vi "SaveTrendData.vi"(6 "registry":T9, 8 "error in (no error)":errorcluster, 9 "data":T13, 10 "data event config":T17, 11 "data event":T1) -> (0 "error out":errorcluster, 3 "data event out":T1)   [LabVIEW 2017, in "EmsaDataEventCreator.lvlib"]
uses:
  <vilib>/addons/InsightCM/Devices/Shared/Emsa/EmsaDataEventCreator/EmsaDataEventCreator.lvlib
  <vilib>/addons/InsightCM/Devices/Shared/Emsa/EmsaDataEventCreator/controls/DataEventConfig.ctl
  <vilib>/addons/PointValueMap/controls/PointMap.ctl
  <vilib>/addons/InsightCM/Devices/Shared/Emsa/EmsaDataEventCreator/controls/SweepParams.ctl
  <vilib>/addons/InsightCM/Devices/Shared/Common/DataFlow/controls/Data.ctl
  <vilib>/addons/InsightCM/Utilities/DataAccessors/controls/wfmSGL_DVR.ctl
  <vilib>/addons/InsightCM/Devices/Shared/Common/DataFlow/controls/Type.ctl
  <vilib>/addons/InsightCM/Devices/Shared/Emsa/EmsaDataEventCreator/controls/Registry.ctl
  <vilib>/addons/InsightCM/Devices/Shared/Emsa/EmsaDataEventCreator/controls/Registry_Sweep.ctl
  <vilib>/addons/InsightCM/Devices/Shared/Common/DataEvent/controls/DataSetType.ctl
  <vilib>/addons/InsightCM/MessageBus/Base/controls/KeyValuePair.ctl
  <vilib>/addons/InsightCM/Devices/Shared/Common/DataEventCreator/controls/Registry_Trend.ctl
  <vilib>/addons/InsightCM/Devices/Shared/Common/DataEvent/controls/Event.ctl
  <vilib>/addons/InsightCM/MessageBus/Base/controls/DataEvent.ctl
  <vilib>/addons/InsightCM/Devices/Shared/Common/DataEvent/controls/DataSet.ctl
  <vilib>/addons/InsightCM/MessageBus/Base/controls/DataSetMetadata.ctl
  <vilib>/addons/InsightCM/MessageBus/Base/controls/TrendPoint.ctl
  <vilib>/addons/InsightCM/MessageBus/Base/controls/TrendAlarmUpdate.ctl
  <vilib>/addons/InsightCM/MessageBus/Base/controls/TrendAlarmTransition.ctl
  <vilib>/addons/PointValueMap/subVIs/Point_Read_double.vi
  <vilib>/addons/PointValueMap/PointValueMap.lvlib
  <vilib>/addons/InsightCM/Devices/Shared/Common/DataFlow/DataFlow.lvlib
  <vilib>/addons/InsightCM/Devices/Shared/Common/DataEventCreator/DataEventCreator.lvlib
  <vilib>/addons/InsightCM/Devices/Shared/Common/DataEvent/DataEvent.lvlib
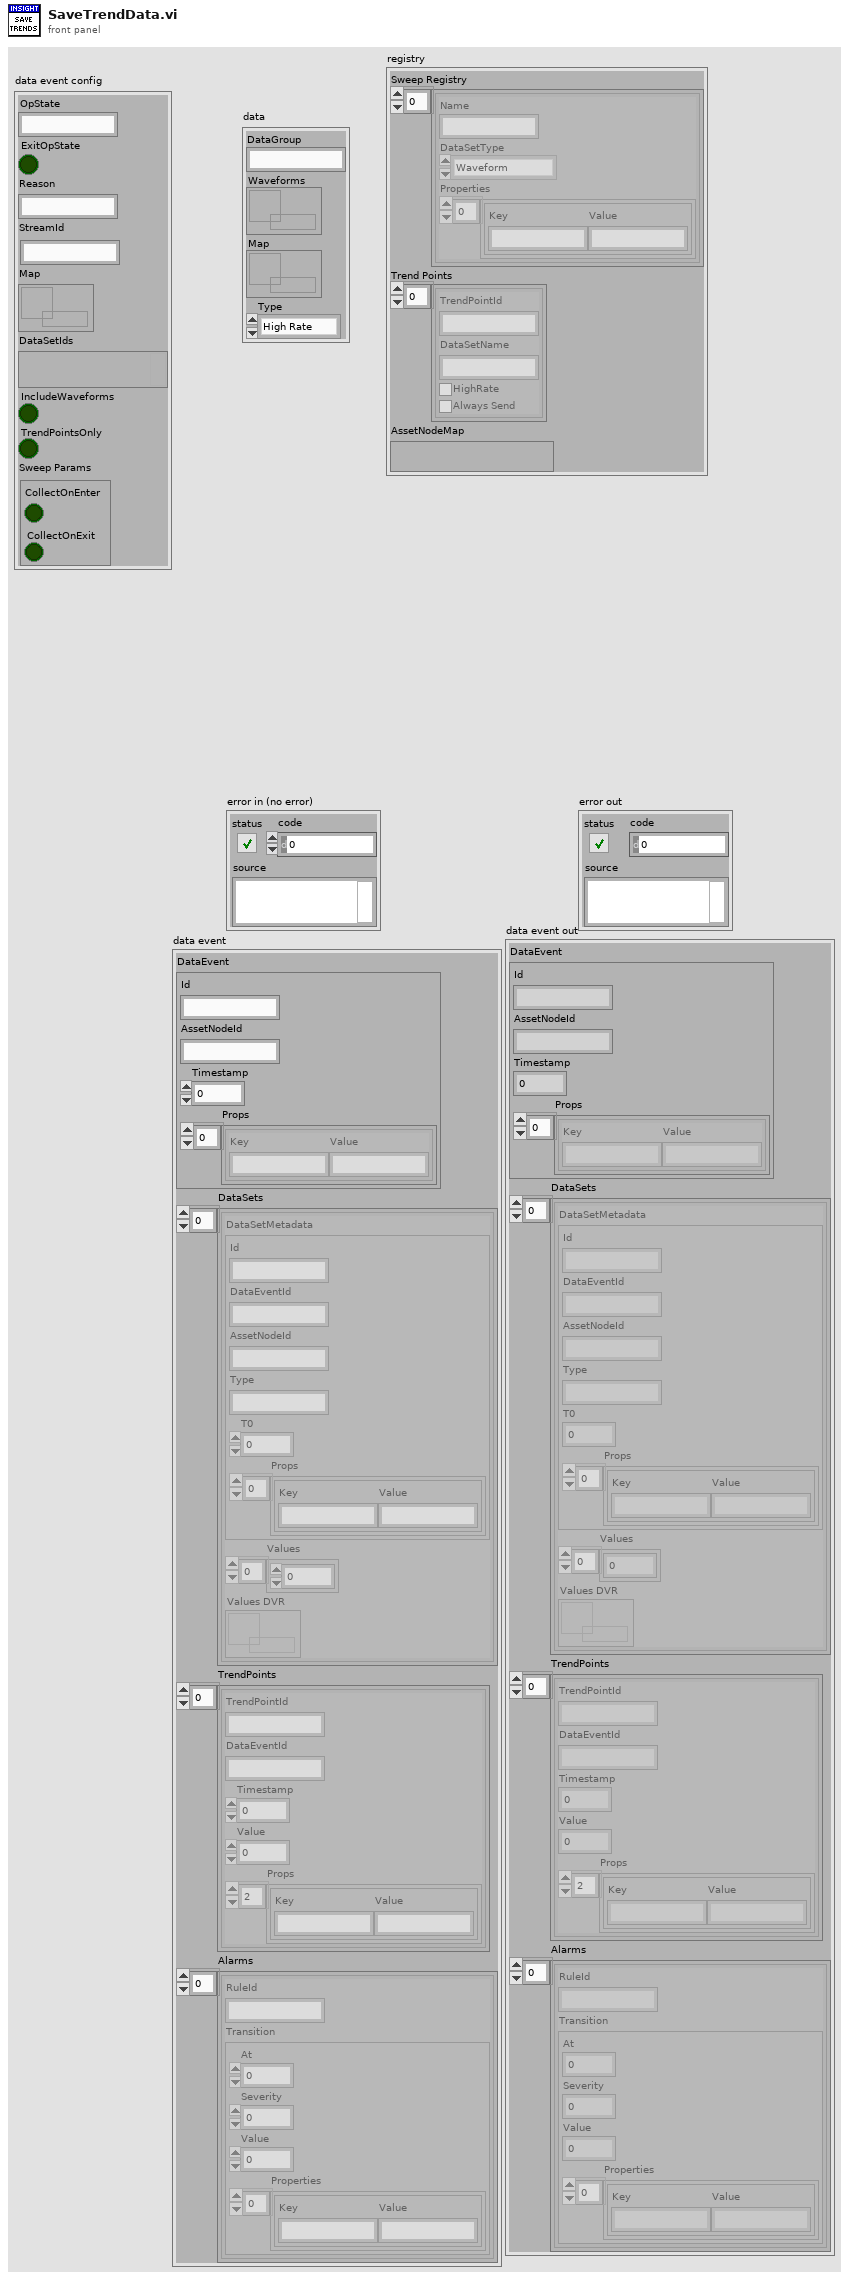
[diagram p1: front panel]
types:
  T1 = typedef "DataEvent.lvlib/Event.ctl" = cluster{"DataEvent":T2, "DataSets":T4[], "TrendPoints":T6[], "Alarms":T7[]}
  T2 = typedef "DataEvent.ctl" = cluster{"Id":string, "AssetNodeId":string, "Timestamp":i64, "Props":T3[]}
  T3 = typedef "KeyValuePair.ctl" = cluster{"Key":string, "Value":string}
  T4 = typedef "DataEvent.lvlib/DataSet.ctl" = cluster{"DataSetMetadata":T5, "Values":sgl[], "Values DVR":refnum<data-value>}
  T5 = typedef "DataSetMetadata.ctl" = cluster{"Id":string, "DataEventId":string, "AssetNodeId":string, "Type":string, "T0":i64, "Props":T3[]}
  T6 = typedef "TrendPoint.ctl" = cluster{"TrendPointId":string, "DataEventId":string, "Timestamp":i64, "Value":dbl, "Props":T3[]}
  T7 = typedef "TrendAlarmUpdate.ctl" = cluster{"RuleId":string, "Transition":T8}
  T8 = typedef "TrendAlarmTransition.ctl" = cluster{"At":i64, "Severity":i32, "Value":dbl, "Properties":T3[]}
  T9 = typedef "EmsaDataEventCreator.lvlib/Registry.ctl" = cluster{"Sweep Registry":T10[], "Trend Points":T12[], "AssetNodeMap":variant}
  T10 = typedef "EmsaDataEventCreator.lvlib/Registry_Sweep.ctl" = cluster{"Name":string, "DataSetType":T11, "Properties":T3[]}
  T11 = typedef "DataEvent.lvlib/DataSetType.ctl" = enum16{"Waveform", "SpeedProfile", "ThermalImage", "EmsaSweep"}
  T12 = typedef "DataEventCreator.lvlib/Registry_Trend.ctl" = cluster{"TrendPointId":string, "DataSetName":string, "HighRate":bool, "Always Send":bool}
  T13 = typedef "DataFlow.lvlib/Data.ctl" = cluster{"DataGroup":string, "Waveforms":T14, "Map":T15, "Type":T16}
  T14 = typedef "wfmSGL_DVR.ctl" = refnum<data-value>
  T15 = typedef "PointValueMap.lvlib/PointMap.ctl" = refnum<data-value>
  T16 = typedef "DataFlow.lvlib/Type.ctl" = enum16{"High Rate", "Low Rate", "Burst Mode"}
  T17 = typedef "EmsaDataEventCreator.lvlib/DataEventConfig.ctl" = cluster{"OpState":string, "ExitOpState":bool, "Reason":string, "StreamId":string, "Map":T15, "DataSetIds":variant, "IncludeWaveforms":bool, "TrendPointsOnly":bool, "Sweep Params":T18}
  T18 = typedef "EmsaDataEventCreator.lvlib/SweepParams.ctl" = cluster{"CollectOnEnter":bool, "CollectOnExit":bool}
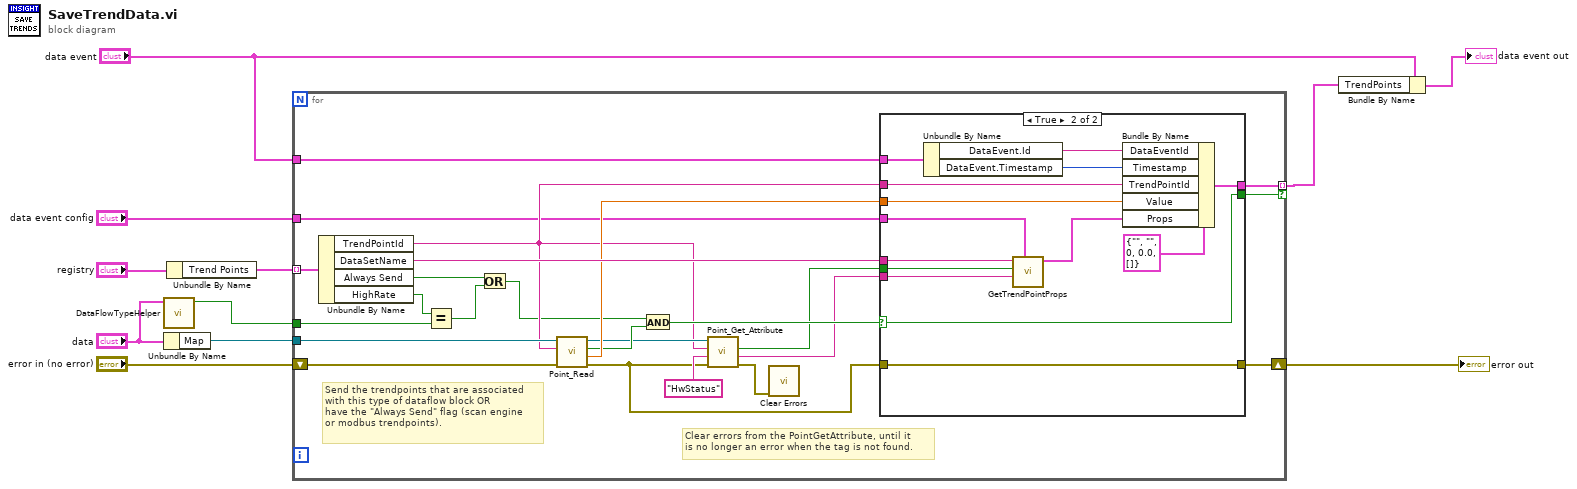
[diagram p0: block diagram]
diagram:
  n1 = call <vilib>:"DataFlowTypeHelper.vi"("data"="data") -> ("high rate"=w1:bool)  [unwired: 8 in, 2 out]
  n2 = Unbundle By Name("data") -> ("Map"=w8:T15)
  n3 = Unbundle By Name("registry") -> ("Trend Points"=w9:T12[])
  n4 = for {
    tunnel: w8 -> [w33]
    tunnel: w9 -> [w32] mode=indexing
    shift-right: [w21] -> w10
    shift-left: "error in (no error)" -> [w34]
    tunnel: "data event" -> [w31]
    tunnel: [w30] -> w4 mode=indexing if=w28
    tunnel: w1 -> [w27]
    tunnel: "data event config" -> [w18]
    # "Clear errors from the PointGetAttribute, until it \nis no longer an error when the tag is not found."
    # "Send the trendpoints that are associated\nwith this type of dataflow block OR\nhave the \"Always Send\" flag (scan engine\nor modbus trendpoints)."
    n5 = Unbundle By Name(w32) -> ("TrendPointId"=w23:string, "DataSetName"=w35:string, "Always Send"=w14:bool, "HighRate"=w15:bool)
    n6 = Equal?(x=w15, y=w27) -> (x = y?=w13:bool)
    n7 = Or(x=w14, y=w13) -> (x .or. y?=w12:bool)
    n8 = call-poly <vilib>:"Point_Read.vi"("Error In"=w34, "Tag"=w23, "Map"=w33) -> ("Error Out"=w16:errorcluster, "Value"=w29:dbl, "Found?"=w26:bool, "Map Out"=w24:T15)  [unwired: 3 in, 2 out]
    n9 = And(x=w12, y=w26) -> (x .and. y?=w25:bool)
    n10 = call <vilib>:"Point_Get_Attribute.vi"("Error In"=w16, "Attribute"="HwStatus", "Tag"=w23, "Map"=w24) -> ("Error Out"=w17:errorcluster, "Value"=w19:string, "Found?"=w20:bool)  [unwired: 4 in, 1 out]
    n11 = call <vilib>:"Clear Errors.vi"("error in (no error)"=w17) -> ()  [unwired: 5 in, 2 out]
    n12 = case shown="True" w25 {
      selector: w25 -> [w37 w42]
      tunnel: w35 -> [_ w51]
      tunnel: w31 -> [_ w50]
      tunnel: [_ w46] -> w30
      tunnel: w29 -> [_ w45]
      tunnel: w23 -> [_ w43]
      tunnel: [w37 w42] -> w28
      tunnel: [w36 w41] -> w21
      tunnel: w16 -> [w36 w41]
      tunnel: w20 -> [_ w40]
      tunnel: w19 -> [_ w38]
      tunnel: w18 -> [_ w39]
      frame False {
      }
      frame True {
        n13 = Unbundle By Name(w50) -> ("DataEvent.Id"=w48:string, "DataEvent.Timestamp"=w47:i64)
        n14 = call <vilib>:"GetTrendPointProps.vi"("data event config"=w39, "hw status"=w38, "found hw status"=w40, "DataSetName"=w51) -> ("key value pairs out"=w44:T3[])  [unwired: 7 in]
        n15 = Bundle By Name(cluster=T6 {"TrendPointId"="", "DataEventId"="", "Timestamp"=0, "Value"=0.0, "Props"=[]} ("TrendPoint"), "DataEventId"=w48, "Timestamp"=w47, "TrendPointId"=w43, "Value"=w45, "Props"=w44) -> (w46:T6)
      }
    }
  }
  "error out" <- w10
  n16 = Bundle By Name(cluster="data event", "TrendPoints"=w4) -> (→"data event out":T1)
